vi "AlazarConfigureRecordAverage.vi"(0 "Handle":u64, 1 "Mode":u32(ring) items=["Disable", "Enable"], 2 "Samples Per Record":u32, 3 "Records Per Average":u32, 4 "Options":u16(ring) items=["Unsigned", "Signed"], 5 "error in (no error)":errorcluster) -> (14 "Handle":u64, 18 "Return Code":u32, 19 "error out":errorcluster)   [LabVIEW 2018]
doc: "This function configures a digitizer to co-add ADC samples from a specified number of records in an accumulator record, and transfer accumulator records rather than the ADC sample values."
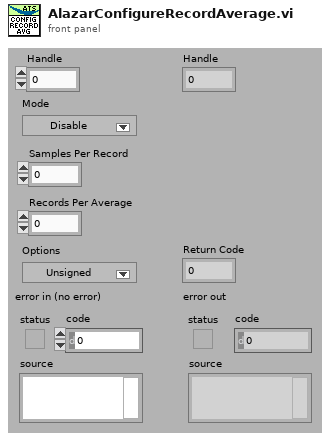
[diagram p1: front panel]
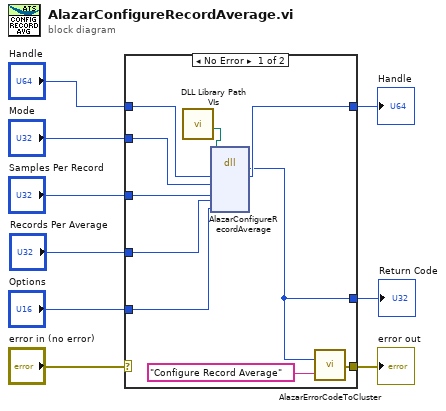
[diagram p0: block diagram]
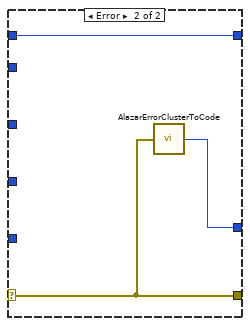
[diagram p2: hidden frame]
diagram:
  n1 = case shown="No Error" "error in (no error)" {
    selector: "error in (no error)" -> [_ w22]
    tunnel: [w13 w22] -> w8
    tunnel: [w12 w21] -> w7
    tunnel: "Handle" -> [w19 w20]
    tunnel: [w18 w20] -> w5
    tunnel: "Mode" -> [w17 _]
    tunnel: "Samples Per Record" -> [w16 _]
    tunnel: "Records Per Average" -> [w15 _]
    tunnel: "Options" -> [w14 _]
    frame No Error {
      n2 = call "DLL Library Path VIs.vi"() -> ("Alazar"=w10:path)  [unwired: 9 in, 2 out]
      n3 = dll-call lib="C:/Project/SerialSectOCT - FFT GPU/SerialSectOCT/Labview Software/DLL/ATSApi.dll" fn="AlazarConfigureRecordAverage"(path in=w10, "handle"=w19, "mode"=w17, "samplesPerRecord"=w16, "recordsPerAverage"=w15, "options"=w14) -> ("return type"=w12:u32, "handle"=w18:u64)  [unwired: 6 in, 2 out]
      n4 = call "AlazarErrorCodeToCluster.vi"("Message"="Configure Record Average", "Error Code"=w12) -> ("error out"=w13:errorcluster)
    }
    frame Error {
      n5 = call "AlazarErrorClusterToCode.vi"("error in (no error)"=w22) -> ("Error Code"=w21:u32)
    }
  }
  "Handle" <- w5
  "error out" <- w8
  "Return Code" <- w7
